vi "Compare DMA Settings.vi"(1 "DMA Settings 2":T1 {"DMA Host Buffer" items=["1 Second"=1, "2 Seconds"=2, "5 Seconds"=5, "10 Seconds"=10]; "dt" format="%#_p"; "Update Rate" items=["1 Hz"=1, "2 Hz"=2, "5 Hz"=5, "10 Hz"=10]}, 2 "DMA Settings 1":T1 {"DMA Host Buffer" items=["1 Second"=1, "2 Seconds"=2, "5 Seconds"=5, "10 Seconds"=10]; "dt" format="%#_p"; "Update Rate" items=["1 Hz"=1, "2 Hz"=2, "5 Hz"=5, "10 Hz"=10]}) -> (0 "equal?":bool)   [LabVIEW 2021, in "FPGA Addon Bitfile Reload Unit Tests.lvclass"]
uses:
  FPGA Addon Bitfile Reload Unit Tests.lvclass
  Addon/Addon Shared/Types/DMA Settings.ctl
  Addon/Addon Shared/Types/Delacing Scheme.ctl
  Addon/Addon Shared/Types/DMA Acquisition Mode.ctl
  Addon/Addon Shared/FPGA Addon Shared.lvlib
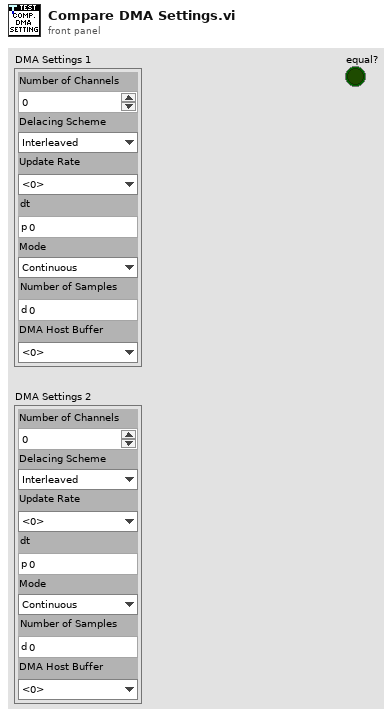
[diagram p1: front panel]
types:
  T1 = typedef "FPGA Addon Shared.lvlib/DMA Settings.ctl" = cluster{"Number of Channels":u8, "Delacing Scheme":T2, "Update Rate":u32, "dt":dbl, "Mode":T3, "Number of Samples":u32, "DMA Host Buffer":u32}
  T2 = typedef "FPGA Addon Shared.lvlib/Delacing Scheme.ctl" = enum8{"Interleaved", "Bitpacked"}
  T3 = typedef "FPGA Addon Shared.lvlib/DMA Acquisition Mode.ctl" = enum8{"Continuous", "Triggered Finite"}
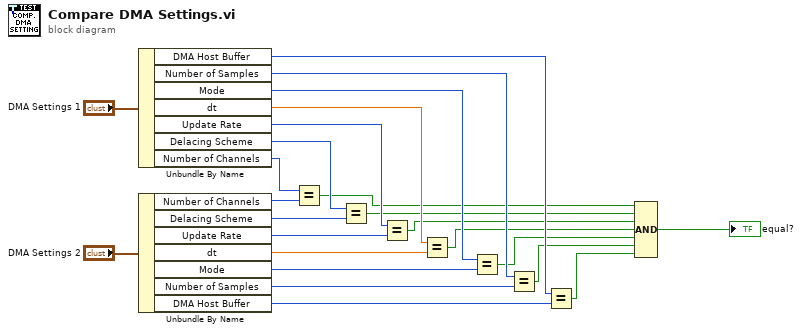
[diagram p0: block diagram]
diagram:
  n1 = Unbundle By Name("DMA Settings 1") -> ("DMA Host Buffer"=w9:u32, "Number of Samples"=w12:u32, "Mode"=w14:T3, "dt"=w16:dbl, "Update Rate"=w18:u32, "Delacing Scheme"=w20:T2, "Number of Channels"=w22:u8)
  n2 = Unbundle By Name("DMA Settings 2") -> ("Number of Channels"=w21:u8, "Delacing Scheme"=w19:T2, "Update Rate"=w17:u32, "dt"=w15:dbl, "Mode"=w13:T3, "Number of Samples"=w11:u32, "DMA Host Buffer"=w10:u32)
  n3 = Equal?(x=w22, y=w21) -> (x = y?=w8:bool)
  n4 = Equal?(x=w20, y=w19) -> (x = y?=w7:bool)
  n5 = Equal?(x=w18, y=w17) -> (x = y?=w6:bool)
  n6 = Equal?(x=w16, y=w15) -> (x = y?=w5:bool)
  n7 = Equal?(x=w14, y=w13) -> (x = y?=w4:bool)
  n8 = Equal?(x=w12, y=w11) -> (x = y?=w3:bool)
  n9 = Equal?(x=w9, y=w10) -> (x = y?=w2:bool)
  n10 = Compound Arithmetic op=AND(w8, w7, w6, w5, w4, w3, w2) -> (→"equal?":bool)
